vi "Call Synchronous.vi"(8 "error in (no error)":errorcluster, 10 "Data In":variant, 11 "VI Path":path) -> (0 "error out":errorcluster, 2 "Data Out":variant)   [LabVIEW 2020]
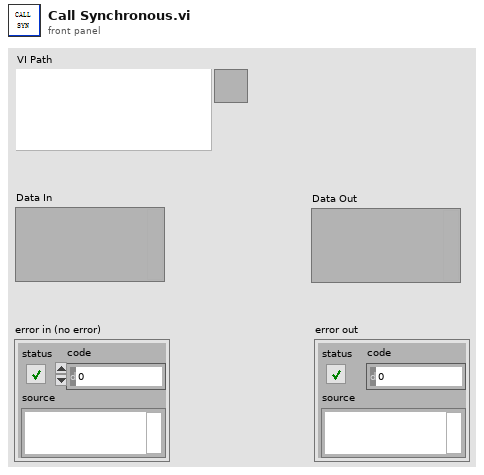
[diagram p1: front panel]
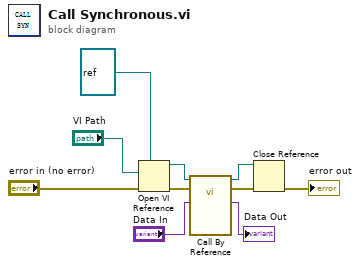
[diagram p0: block diagram]
diagram:
  n1 = Open VI Reference(type specifier VI Refnum (for type only)=refnum<vi> refnum, vi path="VI Path", error in (no error)="error in (no error)") -> (vi reference=w10:refnum<vi>, error out=w9:errorcluster)  [unwired: 3 in]
  n2 = call-by-ref "?"(reference=w10, error in=w9, "Data In"="Data In") -> (reference out=w2:refnum<vi>, error out=w3:errorcluster, "Data Out"=→"Data Out":variant)  [unwired: 10 in]
  n3 = Close Reference(reference=w2, error in (no error)=w3) -> (error out=→"error out":errorcluster)
